vi "Memory Delete Location.vi"(8 "error in (no error)":errorcluster, 10 "Location":i16=1 min=1 max=99 step=1, 11 "VISA resource name":refnum<visa-resource-name>) -> (0 "error out":errorcluster, 3 "VISA resource name out":refnum<visa-resource-name>)   [LabVIEW 2025, in "Chroma 19572.lvlib"]
uses:
  <instrlib>/Chroma 19572/Chroma 19572.lvlib
panel:
  # "Memory: Delete Location"
  # "1...99"
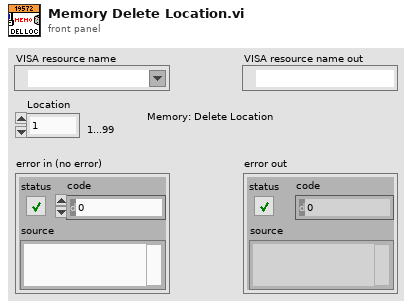
[diagram p1: front panel]
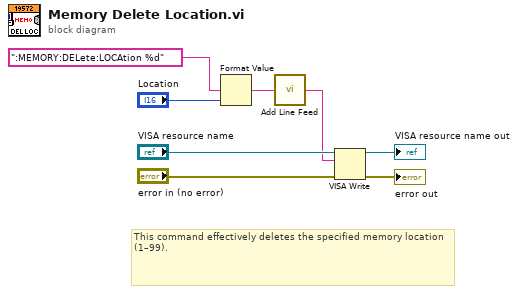
[diagram p0: block diagram]
diagram:
  # "This command effectively deletes the specified memory location (1–99)."
  n1 = Format Value(format string=":MEMORY:DELete:LOCAtion %d", value (0)="Location") -> (output string=w3:string)  [unwired: 1 in]
  n2 = call <instrlib>:"Add Line Feed.vi"("Command string"=w3) -> ("Concatenated string"=w1:string)  [unwired: 4 in]
  n3 = VISA Write(VISA resource name="VISA resource name", write buffer=w1, error in (no error)="error in (no error)") -> (VISA resource name out=→"VISA resource name out":refnum<visa-resource-name>, error out=→"error out":errorcluster)  [unwired: 1 out]
